vi "motor driver -- wrapper.vi"(6 "Instrument Address":refnum<visa-resource-name>="ASRL2::INSTR", 7 "stepper driver action":T2, 10 "speed IN":dbl, 11 "number IN":dbl format="%#_13g") -> (1 "stepper motor state OUT":T1, 2 "speed OUT":dbl, 3 "number OUT":dbl)   [LabVIEW 2018]
uses:
  stepper driver action.ctl
  stepper motor state.ctl
  motor type.ctl
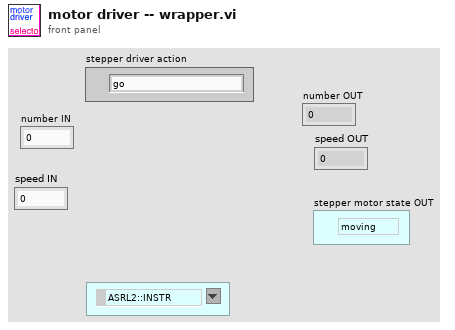
[diagram p1: front panel]
types:
  T1 = typedef "stepper motor state.ctl" = enum16{"moving", "stopped"}
  T2 = typedef "stepper driver action.ctl" = enum16{"go", "void", "stop", "check", "init", "sync", "set", "set speed", "--check status", "--check value"}
  T3 = typedef "motor type.ctl" = enum16{"IMS", "BLM"}
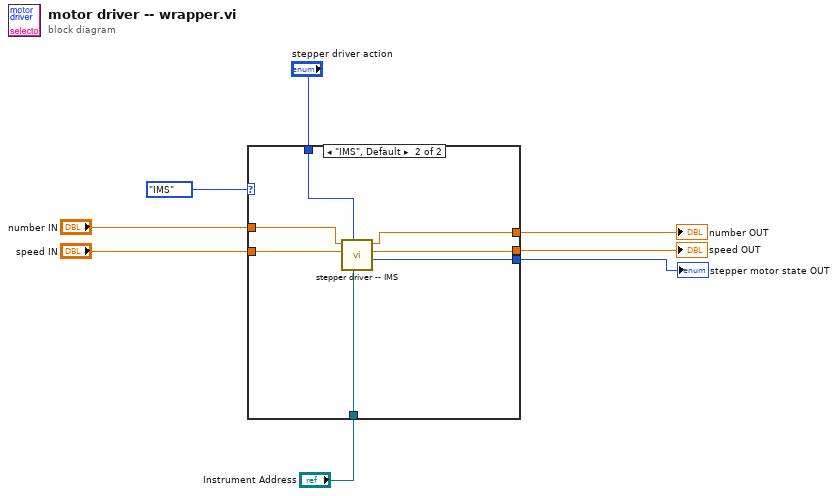
[diagram p0: block diagram]
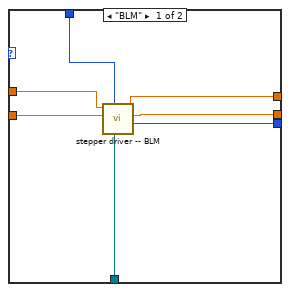
[diagram p2: hidden frame]
diagram:
  n1 = case shown="\"IMS\", Default" motor_type."IMS" ("motor selector") {
    tunnel: "stepper driver action" -> [w15 w22]
    tunnel: [w14 w21] -> w6
    tunnel: [w13 w20] -> w5
    tunnel: [w12 w19] -> w4
    tunnel: "number IN" -> [w11 w18]
    tunnel: "speed IN" -> [w10 w17]
    tunnel: "Instrument Address" -> [w9 w16]
    frame "BLM" {
      n2 = call "stepper driver -- BLM.vi"("Instrument Address"=w9, "stepper driver action"=w15, "speed IN"=w10, "number"=w11) -> ("stepper motor state OUT"=w13:T1, "speed"=w14:dbl, "number out"=w12:dbl)  [unwired: 5 in]
    }
    frame "IMS", Default {
      n3 = call "stepper driver -- IMS.vi"("Instrument Address"=w16, "stepper driver action"=w22, "speed IN"=w17, "number"=w18) -> ("stepper motor state OUT"=w20:T1, "speed"=w21:dbl, "number out"=w19:dbl)  [unwired: 5 in]
    }
  }
  "speed OUT" <- w6
  "stepper motor state OUT" <- w5
  "number OUT" <- w4
